vi "Init Module.vi"(8 "error in (no error)":errorcluster, 10 "Close Master Reference (F)":bool, 11 "Cloneable Module Admin in":refnum<class "Delacor_lib_QMH_Cloneable Module Admin.lvclass">) -> (0 "error out":errorcluster, 2 "Client HTTP Get Request Events":T1, 3 "Cloneable Module Admin out":refnum<class "Delacor_lib_QMH_Cloneable Module Admin.lvclass">)   [LabVIEW 2020, in "Client HTTP Get.lvlib"]
doc: "Initialize the module by creating Broadcast Events, Request Events, and synchronization rendezvous. Also, since this is a cloneable module, add it to the cloneable registry and update the Module Admin class.\n\nSee the block diagram for an explanation of the 'Close Master Reference' parameter.\n_____\nBased on DQMH Project Template 6.0.0.91."
uses:
  Client HTTP Get.lvlib
  <vilib>/Delacor/Delacor QMH/Libraries/Cloneable Module Admin_class/Delacor_lib_QMH_Cloneable Module Admin.lvclass
  C:/Program Files (x86)/National Instruments/LabVIEW 2020/vi.lib/Delacor/Delacor QMH/Libraries/Module Admin_class/Delacor_lib_QMH_Module Admin.lvclass
  Request Events--cluster.ctl
  Stop Argument--cluster.ctl
  Do Something Argument--cluster.ctl
  Do Something Else Argument--cluster.ctl
  Do Something Else and Wait for Reply Argument--cluster.ctl
  Do Something Else and Wait (Reply Payload)--cluster.ctl
  Show Panel Argument--cluster.ctl
  Hide Panel Argument--cluster.ctl
  Show Diagram Argument--cluster.ctl
  Get Module Execution Status Argument--cluster.ctl
  <vilib>/Delacor/Delacor QMH/Libraries/Module Admin_class/Delacor_lib_QMH_Module Admin.lvclass/Delacor_lib_QMH_Module Admin.ctl
  <vilib>/Delacor/Delacor QMH/Libraries/Cloneable Module Admin_class/Delacor_lib_QMH_Cloneable Module Admin.lvclass/Delacor_lib_QMH_Cloneable Module Admin.ctl
  <vilib>/Delacor/Delacor QMH/Libraries/Module Admin_class/Delacor_lib_QMH_Get External Launch.vi
  <vilib>/Delacor/Delacor QMH/Libraries/Cloneable Module Admin_class/Delacor_lib_QMH_Get Module ID.vi
  <vilib>/Delacor/Delacor QMH/Libraries/Cloneable Module Admin_class/Delacor_lib_QMH_Set Close Master Reference.vi
  <vilib>/Delacor/Delacor QMH/Libraries/Cloneable Module Admin_class/Delacor_lib_QMH_Set First.vi
  Clone Registration/Clone Registration.lvlib
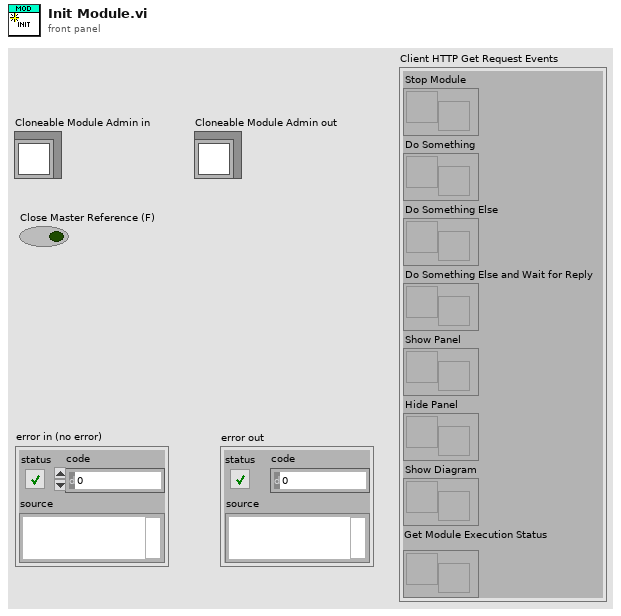
[diagram p1: front panel]
types:
  T1 = typedef "Client HTTP Get.lvlib/Request Events--cluster.ctl" = cluster{"Stop Module":refnum<user-event>, "Do Something":refnum<user-event>, "Do Something Else":refnum<user-event>, "Do Something Else and Wait for Reply":refnum<user-event>, "Show Panel":refnum<user-event>, "Hide Panel":refnum<user-event>, "Show Diagram":refnum<user-event>, "Get Module Execution Status":refnum<user-event>}
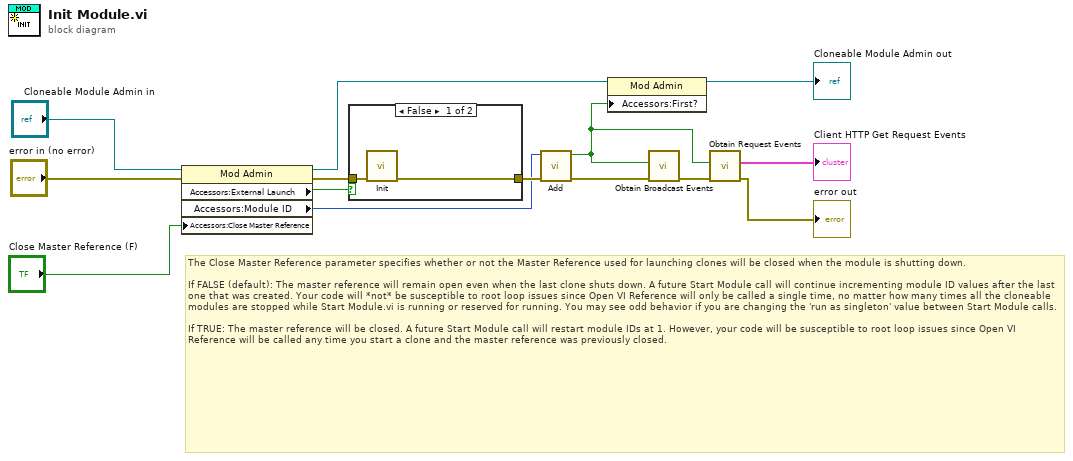
[diagram p0: block diagram]
diagram:
  # "The Close Master Reference parameter specifies whether or not the Master Reference used for launching clones will be closed when the module is shutting down. \n\nIf FALSE (default): The master reference will remain open even when the last clone shuts down. A future Start Module call will continue incrementing module ID values after the last one that was created. Your code will *not* be susceptible to root loop issues since Open VI Reference will only be called a single time, no matter how many times all the cloneable modules are stopped while Start Module.vi is running or reserved for running. You may see odd behavior if you are changing the 'run as singleton' value between Start Module calls.\n\nIf TRUE: The master reference will be closed. A future Start Module call will restart module IDs at 1. However, your code will be susceptible to root loop issues since Open VI Reference will be called any time you start a clone and the master reference was previously closed."
  n1 = property class="Mod Admin"(reference="Cloneable Module Admin in", error in="error in (no error)", "Accessors:Close Master Reference"="Close Master Reference (F)") -> (reference out=w8:refnum<class "Delacor_lib_QMH_Cloneable Module Admin.lvclass">, error out=w3:errorcluster, "Accessors:External Launch"=w7:bool, "Accessors:Module ID"=w2:i32)
  n2 = case "External Launch?" shown="False" w7 {
    tunnel: [w16 w17] -> w13
    tunnel: w3 -> [w15 w17]
    frame False {
      n3 = call "Init.vi"("error in (no error)"=w15) -> ("error out"=w16:errorcluster)  [unwired: 7 in, 3 out]
    }
    frame True {
      # "Init of Clone's registration\nhappened at Start Module.vi"
    }
  }
  n4 = call "Add.vi"("error in (no error)"=w13, "Module ID"=w2) -> ("error out"=w14:errorcluster, "First?"=w9:bool)  [unwired: 7 in, 1 out]
  n5 = property class="Mod Admin"(reference=w8, "Accessors:First?"=w9) -> (reference out=→"Cloneable Module Admin out":refnum<class "Delacor_lib_QMH_Cloneable Module Admin.lvclass">)  [unwired: 1 in, 1 out]
  n6 = call "Obtain Broadcast Events.vi"("error in (no error)"=w14, "Create New? (F)"=w9) -> ("error out"=w12:errorcluster)  [unwired: 8 in, 1 out]
  n7 = call "Obtain Request Events.vi"("error in (no error)"=w12, "Create New? (F)"=w9) -> ("error out"=→"error out":errorcluster, "Client HTTP Get Request Events"=→"Client HTTP Get Request Events":T1)  [unwired: 8 in]
